vi "New-stim indicator.vi"(11 "array":dbl[](array[numeric])) -> (3 "indicator":cluster{u32, u32}[](array[cluster]))   [LabVIEW 2019]
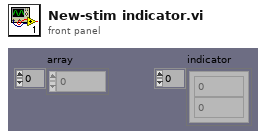
[diagram p1: front panel]
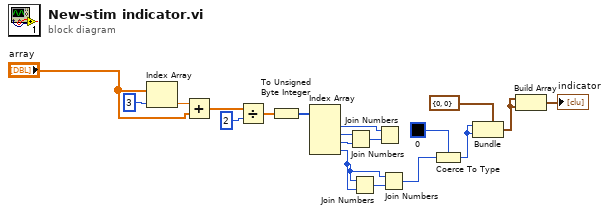
[diagram p0: block diagram]
diagram:
  n1 = Index Array(array="array", index=3) -> (element=w7:dbl)
  n2 = Add(x=w7, y="array") -> (x+y=w8:dbl[])
  n3 = Divide(x=w8, y=2 ("index")) -> (x/y=w10:dbl[])
  n4 = To Unsigned Byte Integer(number=w10) -> (unsigned 8bit integer=w11:u8[])
  n5 = Index Array(array=w11) -> (element #1=w16:u8, element #2=w17:u8, element #3=w18:u8, element #4=w2:u8)  [unwired: 4 in]
  n6 = Join Numbers(hi=w17, lo=w18) -> ((hi.lo)=w15:u16)
  n7 = Join Numbers(hi=w2, lo=w2) -> ((hi.lo)=w3:u16)
  n8 = Join Numbers(hi=w16, lo=w15) -> ()  [unwired: 1 out]
  n9 = Join Numbers(hi=w2, lo=w3) -> ((hi.lo)=w1:u32)
  n10 = Coerce To Type(0:w1, 1:u32 0) -> (2:w14:u32)
  n11 = Bundle(cluster=cluster{u32, u32} {0, 0}, w14, w14) -> (w4:cluster{u32, u32})
  n12 = Build Array(w4, w4) -> (→"indicator":cluster{u32, u32}[])
